vi "Mapping v10.6.1.vi"(5 "Simulate Spectra":bool, 7 "Simulate Drive":bool) -> ()   [LabVIEW 2010]
uses:
  TypeDefs/Mapping Spectra Params.ctl
  TypeDefs/Mapping Drive Params v10.6.0.ctl
  NPC3SG/TypeDefs/NPC3SG Set Positions.ctl
  NPC3SG/TypeDefs/NPC3SG Current Values.ctl
  iHR550/TypeDefs/iHR Current Values.ctl
  ITC503/TypeDefs/ITC503 Current Values.ctl
  TypeDefs/Mapping Input Parameters v10.6.0.ctl
  Symphony/TypeDefs/Symphony Area Format.ctl
  <vilib>/Utility/miscctls.llb/LVPointTypeDef.ctl
  Global Variables.vi
panel:
  in  "Input Parameters":T1={"Drive Connection Port"="", "ITC503 Current Values"={"ITC503 Heater"=0.0, "ITC503 Temperature"=0.0, "ITC503 P"=0.0, "ITC503 I"=0.0, "ITC503 D"=0.0, "ITC503 Setpoint"=0.0, "ITC503 Gradient"=0.0, "ITC503 Heater Auto"=FALSE, "ITC503 PID Auto"=FALSE}, "Wavelengths (nm)"=[], "Drive Current Values"={"Drive X Position"=0.0, "Drive Y Position"=0.0, "Drive Z Position"=0.0}, "iHR Current Values"={"iHR 550 Front Entrance"=0.0, "iHR550 Side Exit"=0.0, "iHR550 Wavelength"=897.9988, "iHR550 Exit Mirror"=2, "iHR550 Grating"="1", "Grating Index"=1}, "Spectra Settings"={"Integration Time"=1.0, "Repetitions"=1, "Mapping Spectra"=TRUE}, "CCD3500 Temperature"=0.0, "Simulate Drive"=FALSE, "Simulate Spectra"=FALSE, "JYCCDLib.IJYCCDReqd"=refnum, "CCD Area"={"XStart"=1, "YStart"=1, "XStop"=2048, "YStop"=512, "XBin"=1, "YBin"=1}, "CCD Gain"=1, "CCD ADC"=0} {"CCD ADC" items=["20 kHz       ", " 1 MHz       ", " 1 MHz Ultra ", "500 kHz Wrap"]; "CCD Gain" items=["High Light", "Best Dynamic Range", "High Sensitivity"]; "ITC503 Current Values"."ITC503 Gradient" format="%.2f"; "ITC503 Current Values"."ITC503 Setpoint" min=-273.0 max=300000.0 step=0.0001 format="%.1f"; "ITC503 Current Values"."ITC503 I" format="%_1f"; "ITC503 Current Values"."ITC503 P" format="%_1f"; "ITC503 Current Values"."ITC503 Temperature" min=0.0 max=1645.0 step=1e-05 format="%.2f"; "ITC503 Current Values"."ITC503 Heater" min=0.0 max=100.0 step=0.01 scale=0.0..100.0; "Drive Current Values"."Drive Z Position" min=-273.0 max=300000.0 step=0.0001 format="%.3f"; "Drive Current Values"."Drive Y Position" min=-273.0 max=300000.0 step=0.0001 format="%.3f"; "Drive Current Values"."Drive X Position" min=-273.0 max=300000.0 step=0.0001 format="%.3f"; "iHR Current Values"."iHR550 Exit Mirror" items=["EntranceMirror", "ExitMirror", "Front", "Side"]; "Spectra Settings"."Repetitions" min=1 max=100 step=1; "Spectra Settings"."Integration Time" min=0.5 max=6000.0 step=1.0 format="%.1f"}
  out "JYCCDLib.IJYCCDReqd":refnum<k7>
  out "AutoClose":bool
  out "ITC503 Temperature":dbl caption="Sample (K)" min=10.0 max=160.0 step=0.1 format="%.3f"
  out "CCD3500 Temperature":dbl caption="CCD (°C)" min=10.0 max=160.0 step=0.1 format="%.1f"
  in  "CCD Current Rep.":string="0/0"
  in  "Pause":bool
  out "Current Position":T3 {"Drive Z Position" min=-273.0 max=300000.0 step=0.0001 format="%.3f"; "Drive Y Position" min=-273.0 max=300000.0 step=0.0001 format="%.3f"; "Drive X Position" min=-273.0 max=300000.0 step=0.0001 format="%.3f"}
  out "Target Position":T7={"Drive X Set"=10.0, "Drive Y Set"=10.0, "Drive Z Set"=10.0} {"Drive X Set" min=10.0 max=160.0 step=0.1 format="%.3f"; "Drive Z Set" min=10.0 max=160.0 step=0.1 format="%.3f"; "Drive Y Set" min=10.0 max=160.0 step=0.1 format="%.3f"}
  out "Progress":u8(slide) max=10 scale=0.0..100.0
  out "Objective Running":bool caption="Obj."
  out "CCD Running":bool caption="CCD"
  in  "Save Map":bool
  in  "Spectra Params":T5={"Integration Time"=10.0, "Repetitions"=10, "Mapping Spectra"=TRUE} {"Repetitions" min=1 max=100 step=1; "Integration Time" min=0.5 max=6000.0 step=1.0 format="%.1f"}
  in  "Drive Settings":refnum<visa-resource-name>
  in  "Z Position":dbl caption="Z (µm)" min=0.0 max=100.0 step=0.1 format="%.1f"
  in  "Mapping Params":T8={"X Start Position"=0.0, "X Stop Position"=10.0, "Y Start Position"=0.0, "Y Stop Position"=10.0, "Step Size"=1.0} {"Step Size" min=0.005 max=20.0 step=0.005 format="%.3f"; "Y Stop Position" min=0.0 max=140.0 step=0.005 format="%.3f"; "Y Start Position" min=0.0 max=140.0 step=0.005 format="%.3f"; "X Stop Position" min=0.0 max=140.0 step=0.005 format="%.3f"; "X Start Position" min=0.0 max=140.0 step=0.005 format="%.3f"}
  in  "Exit":bool
  out "Measuring":bool
  in  "Start":bool
  out "Filename":string
  out "Full Data":dbl[][](array[numeric])
  out "Live Data":dbl[][](array[numeric])
  in  "ITC503 Current Values":T2 {"ITC503 Gradient" format="%.2f"; "ITC503 Setpoint" min=-273.0 max=300000.0 step=0.0001 format="%.1f"; "ITC503 I" format="%_1f"; "ITC503 P" format="%_1f"; "ITC503 Temperature" min=0.0 max=1645.0 step=1e-05 format="%.2f"; "ITC503 Heater" min=0.0 max=100.0 step=0.01 scale=0.0..100.0}
  in  "iHR Current Values":T4={"iHR 550 Front Entrance"=0.0, "iHR550 Side Exit"=0.0, "iHR550 Wavelength"=897.9988, "iHR550 Exit Mirror"=2, "iHR550 Grating"="1", "Grating Index"=1} {"iHR550 Exit Mirror" items=["EntranceMirror", "ExitMirror", "Front", "Side"]}
  in  "Wavelengths (nm)":dbl[](array[numeric])
  # "Status"
  # "Active"
  # "Target"
  # "Current"
  # "Parameters"
  # "Spectral"
  # "Spectral / Video Mapping"
  # "Mapping"
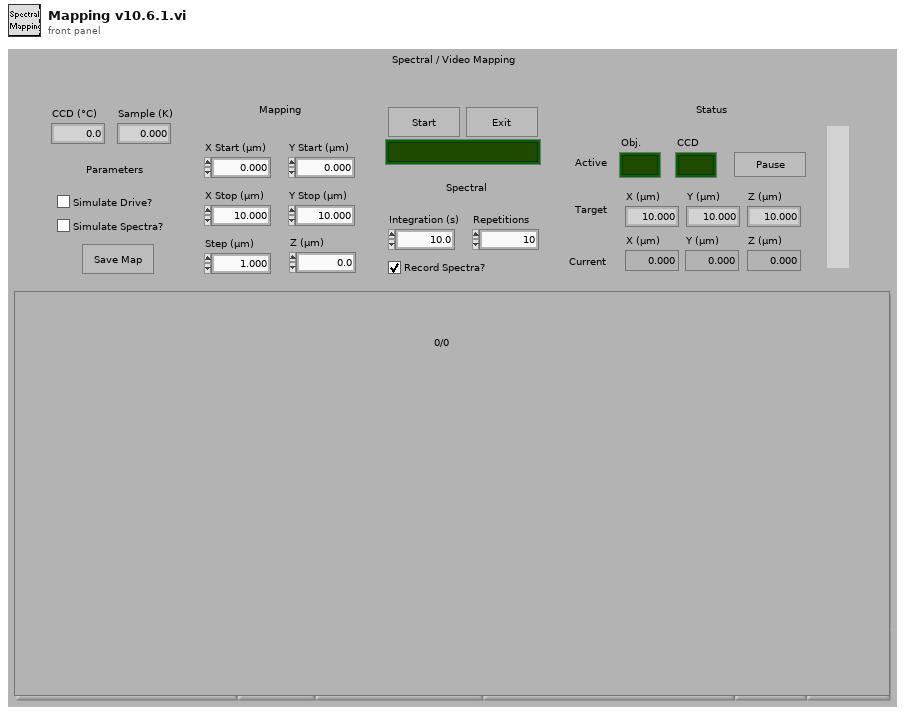
[diagram p1: front panel]
types:
  T1 = typedef "Mapping Input Parameters v10.6.0.ctl" = cluster{"Drive Connection Port":refnum<visa-resource-name>, "ITC503 Current Values":T2, "Wavelengths (nm)":dbl[], "Drive Current Values":T3, "iHR Current Values":T4, "Spectra Settings":T5, "CCD3500 Temperature":dbl, "Simulate Drive":bool, "Simulate Spectra":bool, "JYCCDLib.IJYCCDReqd":refnum<k7>, "CCD Area":T6, "CCD Gain":u16, "CCD ADC":u16}
  T2 = typedef "ITC503 Current Values.ctl" = cluster{"ITC503 Heater":dbl, "ITC503 Temperature":dbl, "ITC503 P":dbl, "ITC503 I":dbl, "ITC503 D":dbl, "ITC503 Setpoint":dbl, "ITC503 Gradient":dbl, "ITC503 Heater Auto":bool, "ITC503 PID Auto":bool}
  T3 = typedef "NPC3SG Current Values.ctl" = cluster{"Drive X Position":dbl, "Drive Y Position":dbl, "Drive Z Position":dbl}
  T4 = typedef "iHR Current Values.ctl" = cluster{"iHR 550 Front Entrance":dbl, "iHR550 Side Exit":dbl, "iHR550 Wavelength":dbl, "iHR550 Exit Mirror":i32, "iHR550 Grating":string, "Grating Index":i32}
  T5 = typedef "Mapping Spectra Params.ctl" = cluster{"Integration Time":dbl, "Repetitions":u16, "Mapping Spectra":bool}
  T6 = typedef "Symphony Area Format.ctl" = cluster{"XStart":i32, "YStart":i32, "XStop":i32, "YStop":i32, "XBin":i32, "YBin":i32}
  T7 = typedef "NPC3SG Set Positions.ctl" = cluster{"Drive X Set":dbl, "Drive Y Set":dbl, "Drive Z Set":dbl}
  T8 = typedef "Mapping Drive Params v10.6.0.ctl" = cluster{"X Start Position":dbl, "X Stop Position":dbl, "Y Start Position":dbl, "Y Stop Position":dbl, "Step Size":dbl}
  T9 = typedef "LVPointTypeDef.ctl" = cluster{"Horizontal":i16, "Vertical":i16}
  T10 = cluster{"Intensities":dbl[], "Wavelengths":dbl[]}[]
  T11 = cluster{"Intensities":dbl[], "Wavelengths":dbl[]}
  T12 = enum32{"invalid app kind", "Development System", "Run Time System", "Student Edition", "Embedded LabVIEW", "Evaluation", "Custom"}
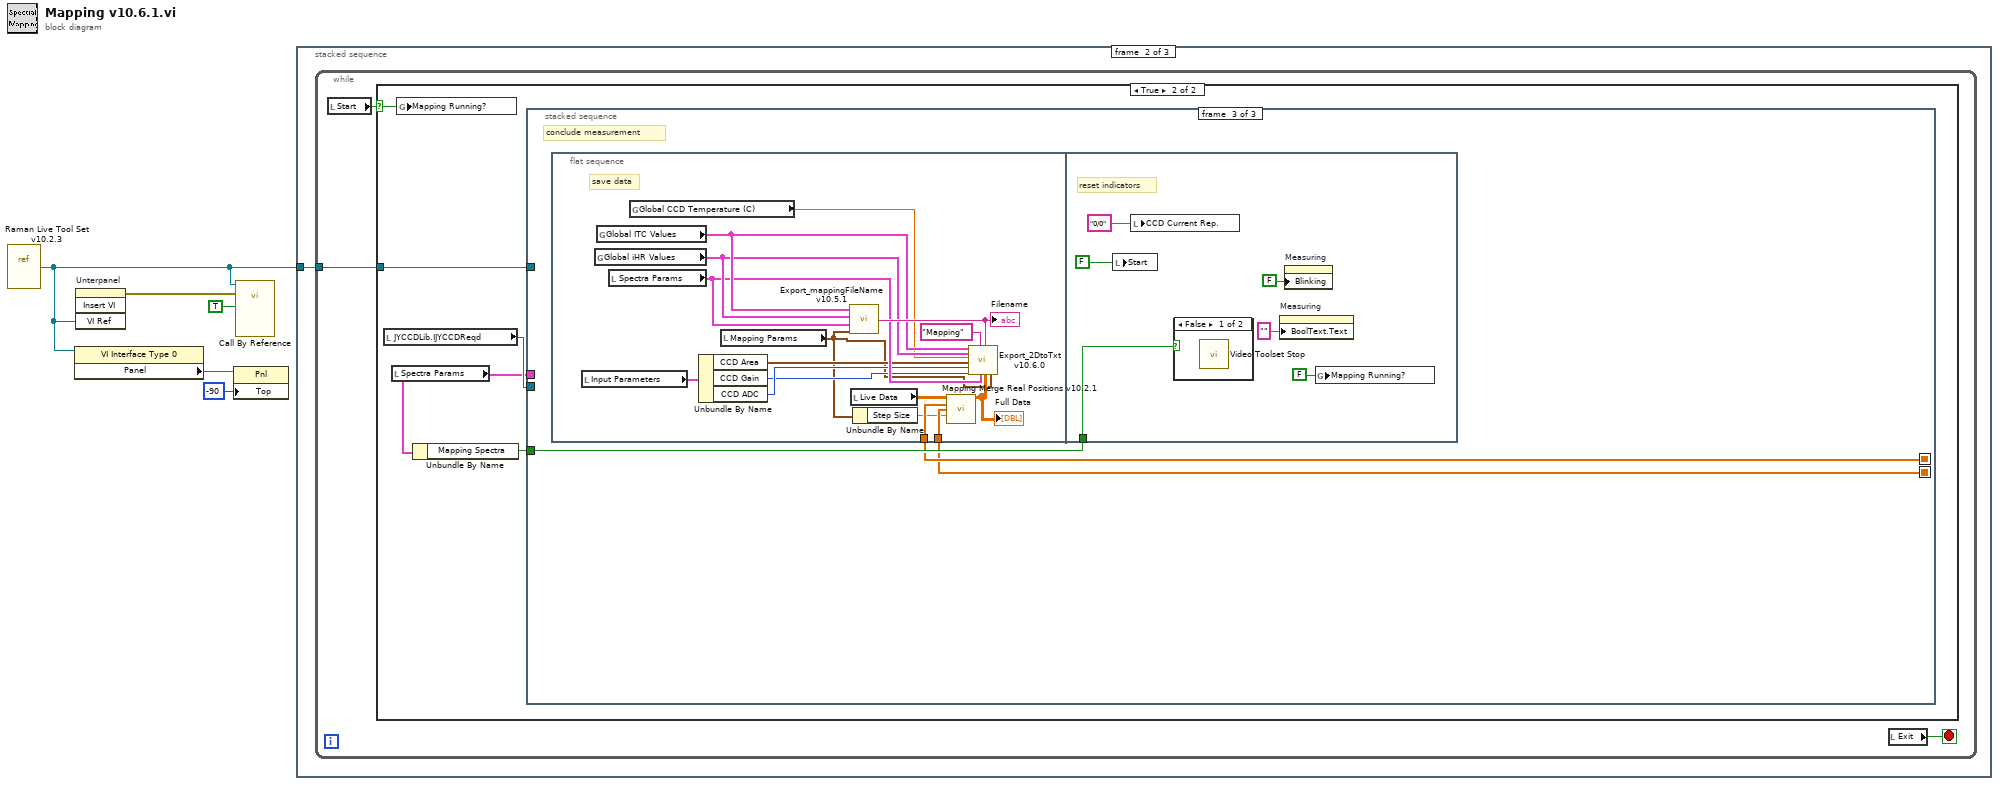
[diagram p0: block diagram]
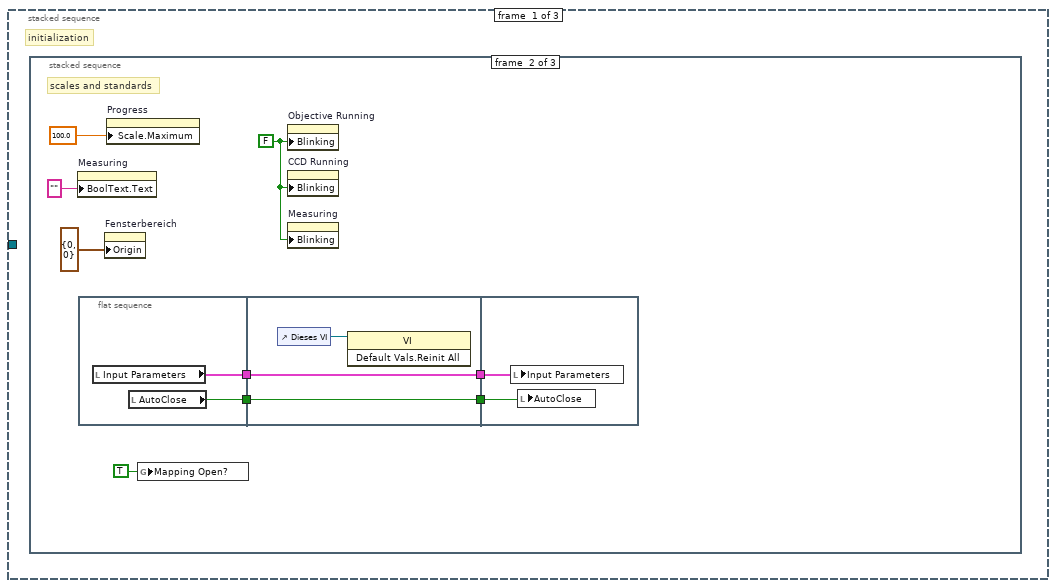
[diagram p2: hidden frame]
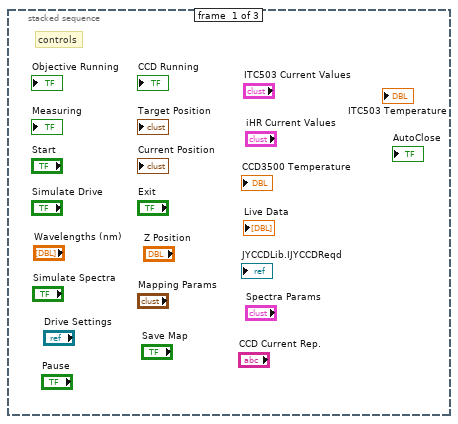
[diagram p3: hidden frame]
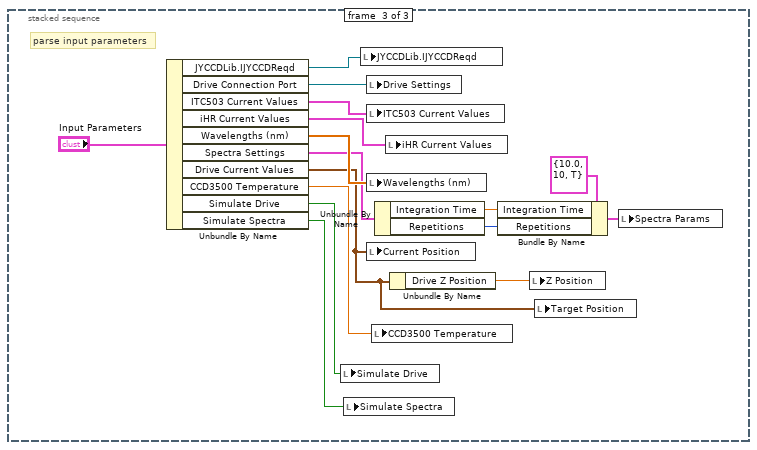
[diagram p4: hidden frame]
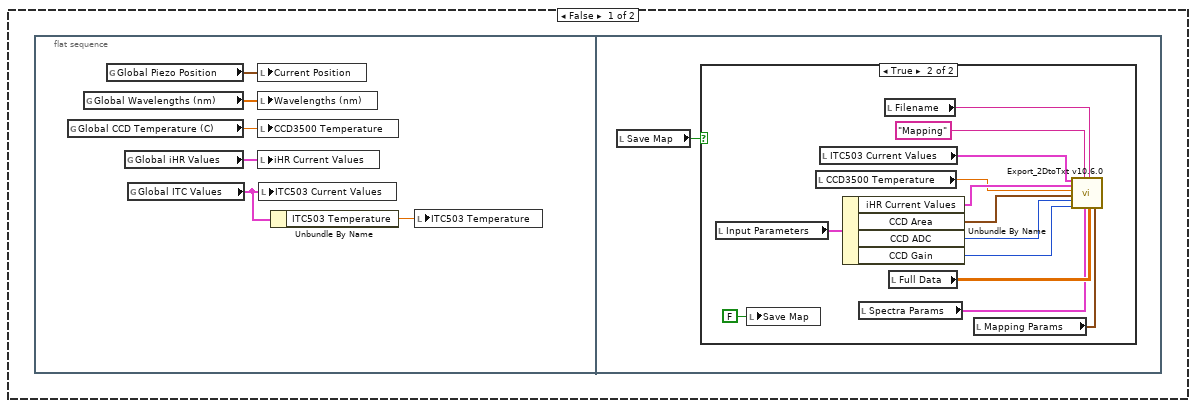
[diagram p5: hidden frame]
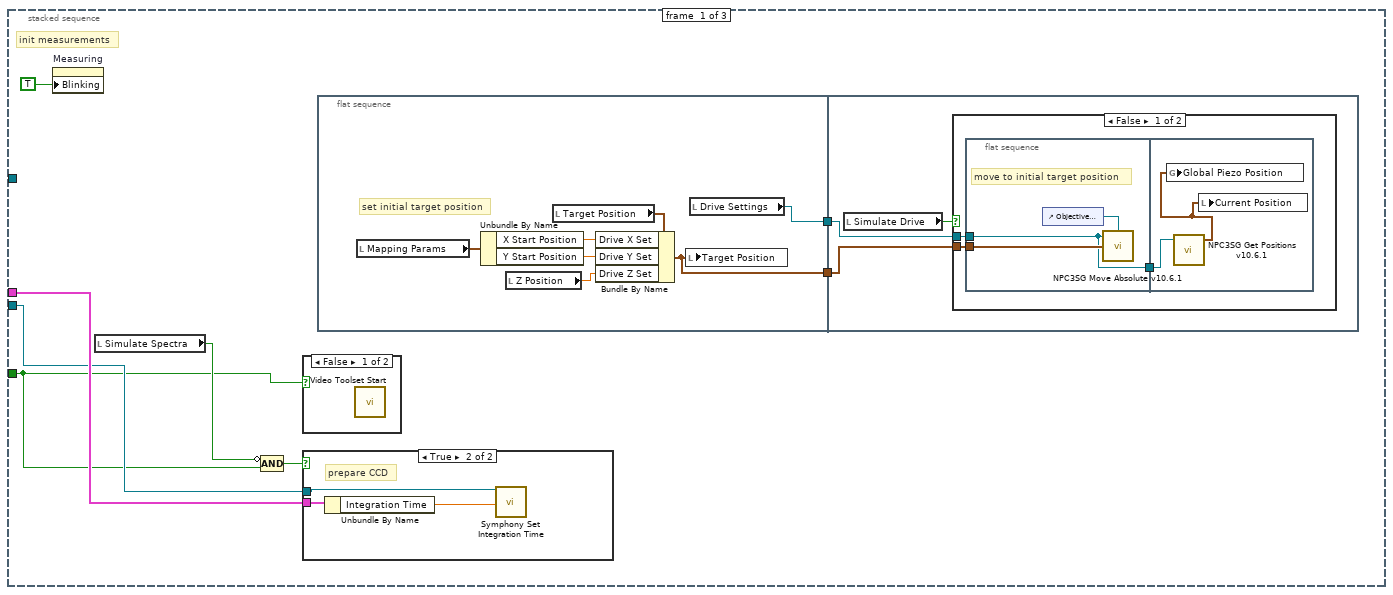
[diagram p7: hidden frame]
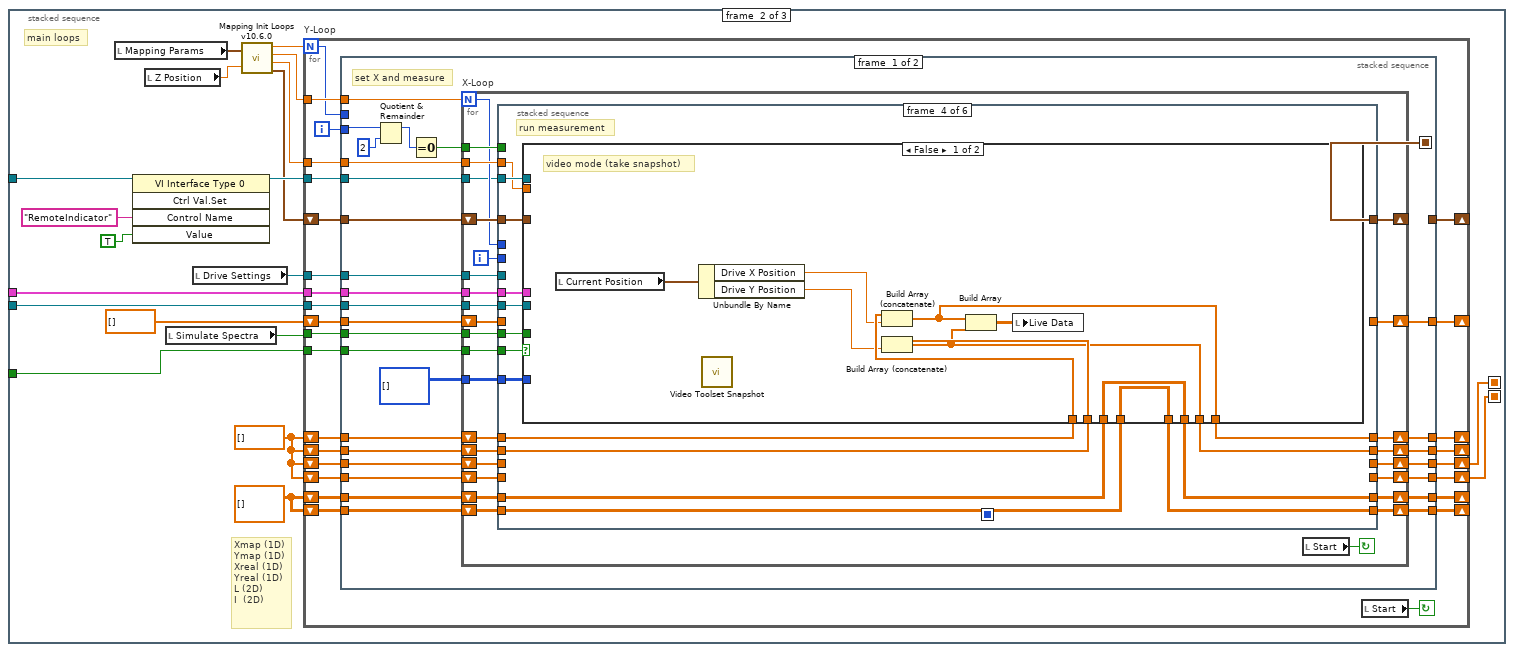
[diagram p11: hidden frame]
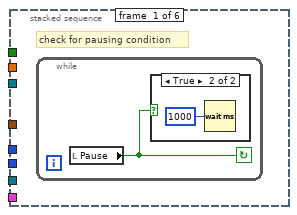
[diagram p12: hidden frame]
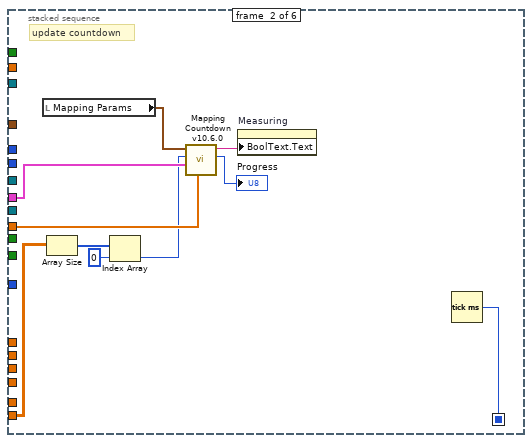
[diagram p14: hidden frame]
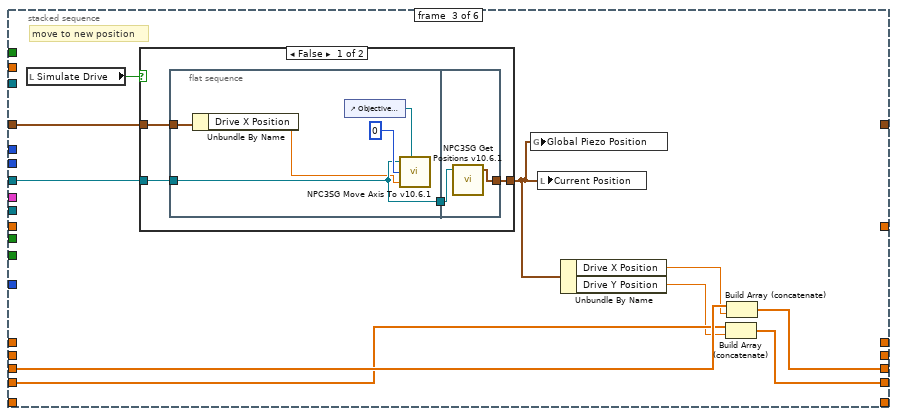
[diagram p15: hidden frame]
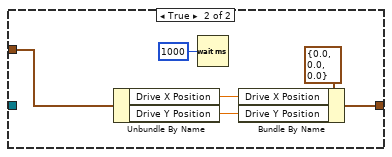
[diagram p16: hidden frame]
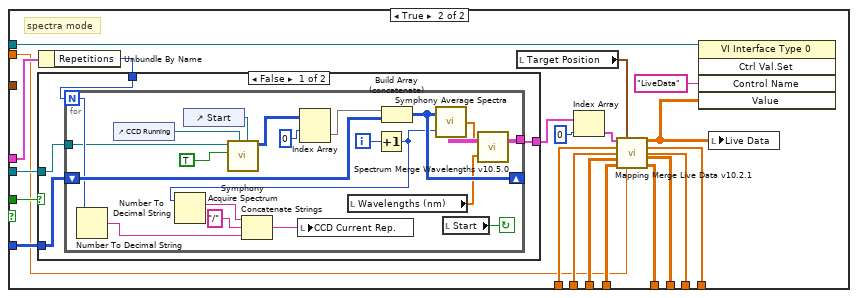
[diagram p17: hidden frame]
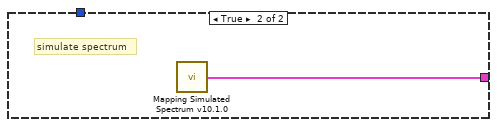
[diagram p18: hidden frame]
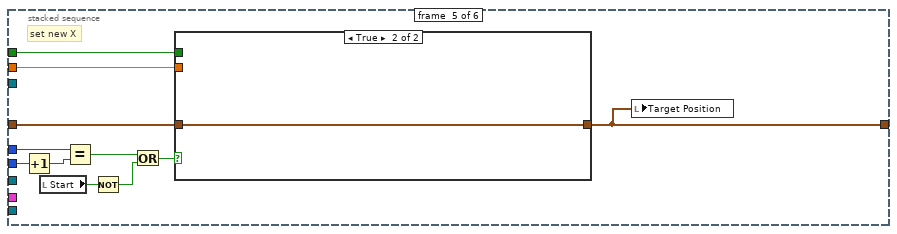
[diagram p19: hidden frame]
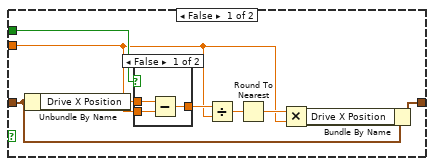
[diagram p20: hidden frame]
diagram:
  n1 = vi-ref "Raman Live Tool Set v10.2.3.vi"() -> (w3:refnum<vi>)
  n2 = property class="VI Interface Type 0"(reference=w3) -> ("Panel"=w2:refnum<vi>)  [unwired: 1 in, 2 out]
  n3 = invoke on="Unterpanel" class="Unterpanel" method="Insert VI"("VI Ref"=w3) -> (error out=w5:errorcluster)  [unwired: 3 in, 3 out]
  n4 = property class="Pnl"(reference=w2, "Top"=-90 ("Position:Oben")) -> ()  [unwired: 1 in, 2 out]
  n5 = call-by-ref "?"(reference=w3, error in=w5, "RemoteIndicator"=TRUE) -> ()  [unwired: 3 in, 2 out]
  n6 = stacked-sequence {
    tunnel: w3 -> [_ w38 w403]
    frame #0 {
      # "initialization"
      n7 = stacked-sequence {
        frame #0 {
          # "controls"
        }
        frame #1 {
          w12 = FALSE ("Blinkend")
          # "scales and standards"
          n8 = property on="Measuring" class="Bool (strict)"("BoolText.Text"="" ("Boolescher Text.Text")) -> ()  [unwired: 2 in, 2 out]
          n9 = flat-sequence {
            tunnel: [w16] -> w9
            tunnel: [w15] -> w6
            tunnel: [w18] -> w10
            tunnel: w9 -> [w18]
            tunnel: [w17] -> w7
            tunnel: w6 -> [w17]
            tunnel: w10 -> [w21]
            tunnel: w7 -> [w20]
            frame #0 {
              n10 = local read "Input Parameters"() -> (w16:T1)
              n11 = local read "AutoClose"() -> (w15:bool)
            }
            frame #1 {
              n12 = control-ref of="Dieses VI"() -> (w19:refnum<vi>)
              n13 = invoke class="VI" method="Default Vals.Reinit All"(reference=w19) -> ()  [unwired: 2 in, 3 out]
            }
            frame #2 {
              n14 = local write "Input Parameters"(w21) -> ()
              n15 = local write "AutoClose"(w20) -> ()
            }
          }
          n16 = property on="Fensterbereich" class="Pane"("Origin"=T9 {"Horizontal"=0, "Vertical"=0}) -> ()  [unwired: 2 in, 2 out]
          n17 = property on="Progress" class="Slide (strict)"("Scale.Maximum"=100.0 ("Skalierung.Bereich:Maximum")) -> ()  [unwired: 2 in, 2 out]
          n18 = global write "Global Variables.vi" "Mapping Open?"(TRUE ("Mapping Open?")) -> ()
          n19 = property on="Objective Running" class="Bool (strict)"("Blinking"=w12) -> ()  [unwired: 2 in, 2 out]
          n20 = property on="CCD Running" class="Bool (strict)"("Blinking"=w12) -> ()  [unwired: 2 in, 2 out]
          n21 = property on="Measuring" class="Bool (strict)"("Blinking"=w12) -> ()  [unwired: 2 in, 2 out]
        }
        frame #2 {
          # "parse input parameters"
          n22 = Unbundle By Name("Input Parameters") -> ("JYCCDLib.IJYCCDReqd"=w24:refnum<k7>, "Drive Connection Port"=w36:refnum<visa-resource-name>, "ITC503 Current Values"=w37:T2, "iHR Current Values"=w27:T4, "Wavelengths (nm)"=w35:dbl[], "Spectra Settings"=w33:T5, "Drive Current Values"=w22:T3, "CCD3500 Temperature"=w28:dbl, "Simulate Drive"=w26:bool, "Simulate Spectra"=w25:bool)
          n23 = local write "Simulate Drive"(w26) -> ()
          n24 = local write "Simulate Spectra"(w25) -> ()
          n25 = local write "JYCCDLib.IJYCCDReqd"(w24) -> ()
          n26 = local write "Drive Settings"(w36) -> ()
          n27 = local write "ITC503 Current Values"(w37) -> ()
          n28 = local write "Wavelengths (nm)"(w35) -> ()
          n29 = local write "Current Position"(w22) -> ()
          n30 = local write "CCD3500 Temperature"(w28) -> ()
          n31 = Unbundle By Name(w33) -> ("Integration Time"=w31:dbl, "Repetitions"=w30:u16)
          n32 = local write "iHR Current Values"(w27) -> ()
          n33 = Unbundle By Name(w22) -> ("Drive Z Position"=w34:dbl)
          n34 = Bundle By Name(cluster=T5 {"Integration Time"=10.0, "Repetitions"=10, "Mapping Spectra"=TRUE} ("Mapping Spectra Settings"), "Integration Time"=w31, "Repetitions"=w30) -> (w29:T5)
          n35 = local write "Z Position"(w34) -> ()
          n36 = local write "Target Position"(w22) -> ()
          n37 = local write "Spectra Params"(w29) -> ()
        }
      }
    }
    frame #1 {
      n38 = while {
        tunnel: w38 -> [w41]
        stop <- w40 stop-if-true
        n39 = local read "Start"() -> (w39:bool)
        n40 = case shown="True" w39 {
          selector: w39 -> [_ w63]
          tunnel: w41 -> [_ w66]
          frame False {
            n41 = flat-sequence {
              frame #0 {
                n42 = global read "Global Variables.vi" "Global CCD Temperature (C)"() -> (w47:dbl)
                n43 = global read "Global Variables.vi" "Global Wavelengths (nm)"() -> (w45:dbl[])
                n44 = global read "Global Variables.vi" "Global Piezo Position"() -> (w46:T3)
                n45 = global read "Global Variables.vi" "Global iHR Values"() -> (w44:T4)
                n46 = global read "Global Variables.vi" "Global ITC Values"() -> (w43:T2)
                n47 = local write "Current Position"(w46) -> ()
                n48 = local write "Wavelengths (nm)"(w45) -> ()
                n49 = local write "CCD3500 Temperature"(w47) -> ()
                n50 = local write "iHR Current Values"(w44) -> ()
                n51 = local write "ITC503 Current Values"(w43) -> ()
                n52 = Unbundle By Name(w43) -> ("ITC503 Temperature"=w42:dbl)
                n53 = local write "ITC503 Temperature"(w42) -> ()
              }
              frame #1 {
                n54 = local read "Save Map"() -> (w48:bool)
                n55 = case shown="True" w48 {
                  frame False {
                  }
                  frame True {
                    n56 = local read "Input Parameters"() -> (w57:T1)
                    n57 = local write "Save Map"(FALSE ("Save Map")) -> ()
                    n58 = local read "CCD3500 Temperature"() -> (w51:dbl)
                    n59 = local read "ITC503 Current Values"() -> (w54:T2)
                    n60 = Unbundle By Name(w57) -> ("iHR Current Values"=w52:T4, "CCD Area"=w53:T6, "CCD ADC"=w56:u16, "CCD Gain"=w55:u16)
                    n61 = local read "Spectra Params"() -> (w50:T5)
                    n62 = local read "Filename"() -> (w60:string)
                    n63 = local read "Full Data"() -> (w58:dbl[][])
                    n64 = local read "Mapping Params"() -> (w49:T8)
                    n65 = call "Export_2DtoTxt v10.6.0.vi"("ITC503 Current Values"=w54, "iHR Current Values"=w52, "CCD Temperature"=w51, "CCD Area"=w53, "CCD ADC"=w56, "CCD Gain"=w55, "Export Type"="Mapping", "Spectra Settings"=w50, "Filename"=w60, "Data (2D)"=w58, "Mapping Parameters"=w49) -> ()  [unwired: 8 in, 1 out]
                  }
                }
              }
            }
          }
          frame True {
            n66 = local read "JYCCDLib.IJYCCDReqd"() -> (w65:refnum<k7>)
            n67 = local read "Spectra Params"() -> (w64:T5)
            n68 = global write "Global Variables.vi" "Mapping Running?"(w63) -> ()
            n69 = Unbundle By Name(w64) -> ("Mapping Spectra"=w62:bool)
            n70 = stacked-sequence {
              seq-local: [_ w96 _] -> [_ _ w378]
              seq-local: [_ w97 _] -> [_ _ w377]
              tunnel: w66 -> [_ w107 _]
              tunnel: w62 -> [w67 w106 w379]
              tunnel: w64 -> [w69 w104 _]
              tunnel: w65 -> [w68 w103 _]
              frame #0 {
                # "init measurements"
                n71 = property on="Measuring" class="Bool (strict)"("Blinking"=TRUE ("Blinkend")) -> ()  [unwired: 2 in, 2 out]
                n72 = local read "Simulate Spectra"() -> (w71:bool)
                n73 = Compound Arithmetic op=AND(invert w71, w67) -> (w70:bool)
                n74 = case shown="False" w67 {
                  frame False {
                    n75 = call "Video Toolset Start.vi"() -> ()  [unwired: 3 in]
                  }
                  frame True {
                  }
                }
                n76 = case shown="True" w70 {
                  tunnel: w68 -> [_ w77]
                  tunnel: w69 -> [_ w76]
                  frame False {
                  }
                  frame True {
                    # "prepare CCD"
                    n77 = Unbundle By Name(w76) -> ("Integration Time"=w75:dbl)
                    n78 = call "Symphony Set Integration Time.vi"("JYCCDLib.IJYCCDReqd"=w77, "Integration (s)"=w75) -> ()  [unwired: 13 in, 1 out]
                  }
                }
                n79 = flat-sequence {
                  tunnel: [w79] -> w73
                  tunnel: [w78] -> w72
                  tunnel: w73 -> [w85]
                  tunnel: w72 -> [w86]
                  frame #0 {
                    # "set initial target position"
                    n80 = local read "Mapping Params"() -> (w84:T8)
                    n81 = Unbundle By Name(w84) -> ("X Start Position"=w82:dbl, "Y Start Position"=w81:dbl)
                    n82 = local read "Z Position"() -> (w80:dbl)
                    n83 = local read "Target Position"() -> (w83:T7)
                    n84 = Bundle By Name(cluster=w83, "Drive X Set"=w82, "Drive Y Set"=w81, "Drive Z Set"=w80) -> (w79:T7)
                    n85 = local write "Target Position"(w79) -> ()
                    n86 = local read "Drive Settings"() -> (w78:refnum<visa-resource-name>)
                  }
                  frame #1 {
                    n87 = local read "Simulate Drive"() -> (w87:bool)
                    n88 = case shown="False" w87 {
                      tunnel: w86 -> [w90 _]
                      tunnel: w85 -> [w88 _]
                      frame False {
                        n89 = flat-sequence {
                          tunnel: w90 -> [w91]
                          tunnel: [w91] -> w89
                          tunnel: w88 -> [w92]
                          tunnel: w89 -> [w94]
                          frame #0 {
                            # "move to initial target position"
                            n90 = control-ref of="Objective Running"() -> (w93:refnum<vi>)
                            n91 = call "NPC3SG Move Absolute v10.6.1.vi"("Running"=w93, "Drive New Abs. Positions"=w92, "Drive Visa Name"=w91) -> ()  [unwired: 2 in]
                          }
                          frame #1 {
                            n92 = call "NPC3SG Get Positions v10.6.1.vi"("Drive Visa Name"=w94) -> ("Drive Current Values"=w95:T3)  [unwired: 6 in]
                            n93 = global write "Global Variables.vi" "Global Piezo Position"(w95) -> ()
                            n94 = local write "Current Position"(w95) -> ()
                          }
                        }
                      }
                      frame True {
                      }
                    }
                  }
                }
              }
              frame #1 {
                w115 = dbl[][] []
                w98 = dbl[] []
                # "main loops"
                # "Xmap (1D)\nYmap (1D)\nXreal (1D)\nYreal (1D)\nL (2D)\nI  (2D)"
                n95 = local read "Mapping Params"() -> (w101:T8)
                n96 = invoke class="VI Interface Type 0" method="Ctrl Val.Set"(reference=w107, "Control Name"="RemoteIndicator" ("Elementname"), "Value"=TRUE) -> (reference out=w109:refnum<vi>)  [unwired: 2 in, 4 out]
                n97 = local read "Z Position"() -> (w100:dbl)
                n98 = local read "Simulate Spectra"() -> (w99:bool)
                n99 = local read "Drive Settings"() -> (w102:refnum<visa-resource-name>)
                n100 = call "Mapping Init Loops v10.6.0.vi"("Z Position"=w100, "Mapping Params"=w101) -> ("Start Positions"=w108:T3, "Step Size"=w110:dbl, "X Steps"=w111:dbl, "Y Steps"=w112:dbl)
                n101 = for "Y-Loop" {
                  N: w112 -> [w128]
                  tunnel: w111 -> [w141]
                  tunnel: w110 -> [w140]
                  shift-right: [w126] -> _
                  shift-left: w108 -> [w127]
                  shift-right: [w132] -> _
                  shift-left: w115 -> [w136]
                  shift-right: [w133] -> _
                  shift-left: w115 -> [w137]
                  shift-right: [w135] -> _
                  shift-left: w98 -> [w139]
                  shift-right: [w134] -> _
                  shift-left: w98 -> [w138]
                  tunnel: w109 -> [w130]
                  tunnel: w99 -> [w129]
                  tunnel: w102 -> [w125]
                  tunnel: w106 -> [w124]
                  tunnel: w104 -> [w123]
                  shift-right: [w121] -> _
                  shift-left: dbl[] [] -> [w122]
                  tunnel: w103 -> [w120]
                  shift-right: [w117] -> w97
                  shift-left: w98 -> [w118]
                  shift-right: [w116] -> w96
                  shift-left: w98 -> [w119]
                  i -> [w131]
                  stop <- w142 continue-if-true
                  n102 = stacked-sequence {
                    seq-local: [w156 _] -> [_ w352]
                    tunnel: w141 -> [w171 _]
                    tunnel: w140 -> [w170 w353]
                    tunnel: w139 -> [w169 _]
                    tunnel: w138 -> [w168 _]
                    tunnel: w137 -> [w167 _]
                    tunnel: w136 -> [w143 _]
                    tunnel: [w166 _] -> w135
                    tunnel: [w165 _] -> w134
                    tunnel: [w164 _] -> w133
                    tunnel: [w163 _] -> w132
                    tunnel: w131 -> [w160 w356]
                    tunnel: w130 -> [w158 _]
                    tunnel: w129 -> [w157 _]
                    tunnel: w128 -> [_ w354]
                    tunnel: w127 -> [w155 _]
                    tunnel: [_ w350] -> w126
                    tunnel: w125 -> [w154 w351]
                    tunnel: w124 -> [w153 _]
                    tunnel: w123 -> [w152 _]
                    tunnel: w122 -> [w151 _]
                    tunnel: [w150 _] -> w121
                    tunnel: w120 -> [w149 _]
                    tunnel: w119 -> [w147 _]
                    tunnel: w118 -> [w146 _]
                    tunnel: [w145 _] -> w117
                    tunnel: [w144 _] -> w116
                    frame #0 {
                      # "set X and measure"
                      n103 = Quotient & Remainder(x=w160, y=2) -> (x-y*floor(x/y)=w161:i32)  [unwired: 1 out]
                      n104 = Equal To 0?(x=w161) -> (x = 0?=w159:bool)
                      n105 = for "X-Loop" {
                        N: w171 -> [w185]
                        tunnel: w170 -> [w197]
                        shift-right: [w196] -> w156
                        shift-left: w155 -> [w198]
                        shift-right: [w191] -> w166
                        shift-left: w169 -> [w195]
                        shift-right: [w190] -> w165
                        shift-left: w168 -> [w194]
                        shift-right: [w188] -> w164
                        shift-left: w167 -> [w193]
                        shift-right: [w189] -> w163
                        shift-left: w143 -> [w192]
                        tunnel: w159 -> [w187]
                        tunnel: w158 -> [w184]
                        tunnel: w157 -> [w183]
                        tunnel: w154 -> [w182]
                        tunnel: w153 -> [w181]
                        tunnel: w152 -> [w180]
                        shift-right: [w179] -> w150
                        shift-left: w151 -> [w178]
                        tunnel: w149 -> [w177]
                        tunnel: u16[][] [] -> [w176]
                        shift-right: [w172] -> w144
                        shift-left: w147 -> [w175]
                        shift-right: [w173] -> w145
                        shift-left: w146 -> [w174]
                        i -> [w186]
                        stop <- w199 continue-if-true
                        n106 = stacked-sequence {
                          seq-local: [_ w206 _ _ _ _] -> [_ _ _ _ _ w341]
                          tunnel: w198 -> [_ _ w221 w254 w318 _]
                          tunnel: w197 -> [_ _ _ w239 w316 _]
                          tunnel: [_ _ _ _ w315 _] -> w196
                          tunnel: w195 -> [_ _ _ w253 _ _]
                          tunnel: w194 -> [_ _ _ w252 _ _]
                          tunnel: w193 -> [_ _ _ w250 _ _]
                          tunnel: w192 -> [_ w205 _ w251 _ _]
                          tunnel: [_ _ _ w249 _ _] -> w191
                          tunnel: [_ _ _ w248 _ _] -> w190
                          tunnel: [_ _ _ w247 _ _] -> w189
                          tunnel: [_ _ _ w246 _ _] -> w188
                          tunnel: w187 -> [_ _ _ _ w317 _]
                          tunnel: w186 -> [_ _ _ _ w321 _]
                          tunnel: w185 -> [_ _ _ _ w319 _]
                          tunnel: w184 -> [_ _ _ w245 _ _]
                          tunnel: w183 -> [_ _ _ w244 _ _]
                          tunnel: w182 -> [_ _ w219 _ _ _]
                          tunnel: w181 -> [_ _ _ w243 _ _]
                          tunnel: w180 -> [_ w208 _ w241 _ _]
                          tunnel: [_ _ _ _ _ w338] -> w179
                          tunnel: w178 -> [_ w207 _ _ _ w340]
                          tunnel: w177 -> [_ _ _ w242 _ _]
                          tunnel: w176 -> [_ _ _ w240 _ _]
                          tunnel: w175 -> [_ _ w218 _ _ _]
                          tunnel: w174 -> [_ _ w217 _ _ _]
                          tunnel: [_ _ w214 _ _ _] -> w173
                          tunnel: [_ _ w213 _ _ _] -> w172
                          frame #0 {
                            # "check for pausing condition"
                            n107 = while {
                              stop <- w200 continue-if-true
                              n108 = local read "Pause"() -> (w200:bool)
                              n109 = case shown="True" w200 {
                                frame False {
                                }
                                frame True {
                                n110 = Wait (ms)(milliseconds to wait=u32 1000) -> ()  [unwired: 1 out]
                                }
                              }
                            }
                          }
                          frame #1 {
                            # "update countdown"
                            n111 = local read "Mapping Params"() -> (w211:T8)
                            n112 = Array Size(array=w205) -> (size(s)=w204:i32[])
                            n113 = Index Array(array=w204, index=0) -> (element=w202:i32)
                            n114 = call "Mapping Countdown v10.6.0.vi"("Execution Times (s)"=w207, "Mapping Spectra Settings"=w208, "Ready Steps"=w202, "Mapping Drive Parameters"=w211) -> ("Progress"=→"Progress":i16, "Time String"=w209:string)  [unwired: 6 in]
                            n115 = property on="Measuring" class="Bool (strict)"("BoolText.Text"=w209) -> ()  [unwired: 2 in, 2 out]
                            n116 = Tick Count (ms)() -> (millisecond timer value=w206:u32)
                          }
                          frame #2 {
                            # "move to new position"
                            n117 = local read "Simulate Drive"() -> (w220:bool)
                            n118 = case shown="False" w220 {
                              tunnel: w221 -> [w225 w237]
                              tunnel: w219 -> [w224 _]
                              tunnel: [w222 w233] -> w212
                              frame False {
                                n119 = flat-sequence {
                                tunnel: w225 -> [w227]
                                tunnel: w224 -> [w228]
                                tunnel: [w228] -> w223
                                tunnel: w223 -> [w232]
                                tunnel: [w231] -> w222
                                frame #0 {
                                n120 = Unbundle By Name(w227) -> ("Drive X Position"=w226:dbl)
                                n121 = control-ref of="Objective Running"() -> (w229:refnum<vi>)
                                n122 = call "NPC3SG Move Axis To v10.6.1.vi"("Drive Visa Name"=w228, "Running"=w229, "Axis"=0, "Drive Set"=w226) -> ()  [unwired: 3 in, 1 out]
                                }
                                frame #1 {
                                n123 = call "NPC3SG Get Positions v10.6.1.vi"("Drive Visa Name"=w232) -> ("Drive Current Values"=w231:T3)  [unwired: 6 in]
                                }
                                }
                              }
                              frame True {
                                n124 = Unbundle By Name(w237) -> ("Drive X Position"=w238:dbl, "Drive Y Position"=w235:dbl)
                                n125 = Wait (ms)(milliseconds to wait=u32 1000 ("Zu wartende ms")) -> ()  [unwired: 1 out]
                                n126 = Bundle By Name(cluster=T3 {"Drive X Position"=0.0, "Drive Y Position"=0.0, "Drive Z Position"=0.0} ("Drive Current Values"), "Drive X Position"=w238, "Drive Y Position"=w235) -> (w233:T3)
                              }
                            }
                            n127 = global write "Global Variables.vi" "Global Piezo Position"(w212) -> ()
                            n128 = local write "Current Position"(w212) -> ()
                            n129 = Unbundle By Name(w212) -> ("Drive X Position"=w216:dbl, "Drive Y Position"=w215:dbl)
                            n130 = Build Array (concatenate)(w217, w215) -> (w214:dbl[])
                            n131 = Build Array (concatenate)(w218, w216) -> (w213:dbl[])
                          }
                          frame #3 {
                            # "run measurement"
                            n132 = case shown="False" w243 {
                              tunnel: w254 -> [_ _]
                              tunnel: w253 -> [w261 w282]
                              tunnel: w252 -> [w260 w281]
                              tunnel: w251 -> [w263 w279]
                              tunnel: w250 -> [w264 w280]
                              tunnel: [w258 w276] -> w249
                              tunnel: [w259 w275] -> w248
                              tunnel: [w263 w278] -> w247
                              tunnel: [w264 w277] -> w246
                              tunnel: w245 -> [_ w284]
                              tunnel: w244 -> [_ w283]
                              tunnel: w242 -> [_ w272]
                              tunnel: w241 -> [_ w271]
                              tunnel: w240 -> [_ w269]
                              tunnel: w239 -> [_ w265]
                              frame False {
                                # "video mode (take snapshot)"
                                n133 = local read "Current Position"() -> (w262:T3)
                                n134 = Unbundle By Name(w262) -> ("Drive X Position"=w257:dbl, "Drive Y Position"=w256:dbl)
                                n135 = call "Video Toolset Snapshot.vi"() -> ()  [unwired: 12 in]
                                n136 = Build Array (concatenate)(w261, w257) -> (w258:dbl[])
                                n137 = Build Array (concatenate)(w260, w256) -> (w259:dbl[])
                                n138 = Build Array(w258, w259) -> (w255:dbl[][])
                                n139 = local write "Live Data"(w255) -> ()
                              }
                              frame True {
                                # "spectra mode"
                                n140 = Unbundle By Name(w271) -> ("Repetitions"=w270:u16)
                                n141 = case shown="False" w283 {
                                tunnel: [w288 w310] -> w268
                                tunnel: w272 -> [w289 _]
                                tunnel: w270 -> [w287 _]
                                tunnel: w269 -> [w286 _]
                                frame False {
                                n142 = for {
                                N: w287 -> [w296]
                                shift-right: [w307] -> _
                                shift-left: w286 -> [w308]
                                tunnel: [w305] -> w288
                                tunnel: w289 -> [w294]
                                i -> [w309]
                                stop <- w303 continue-if-true
                                n143 = Number To Decimal String(number=w296) -> (decimal integer string=w299:string)  [unwired: 1 in]
                                n144 = control-ref of="CCD Running"() -> (w302:refnum<vi>)
                                n145 = control-ref of="Start"() -> (w301:refnum<vi>)
                                n146 = call "Symphony Acquire Spectrum.vi"("Acquire"=w301, "Running"=w302, "ShutterOpen"=TRUE, "JYCCDLib.IJYCCDReqd"=w294) -> ("Raw Data"=w291:i32[][])  [unwired: 6 in, 1 out]
                                n147 = Index Array(array=w291, index (row)=0) -> (element=w290:i32[])  [unwired: 1 in]
                                n148 = local read "Wavelengths (nm)"() -> (w304:dbl[])
                                n149 = Increment(x=w309) -> (x+1=w295:i32)
                                n150 = Number To Decimal String(number=w295) -> (decimal integer string=w298:string)  [unwired: 1 in]
                                n151 = Concatenate Strings(w298, "/" ("string"), w299) -> (w297:string)
                                n152 = local write "CCD Current Rep."(w297) -> ()
                                n153 = Build Array (concatenate)(w290, w308) -> (w307:i32[][])
                                n154 = call "Symphony Average Spectra.vi"("Repetitions"=w295, "Raw Spectra"=w307) -> ("Raw Spectrum"=w306:dbl[])
                                n155 = local read "Start"() -> (w303:bool)
                                n156 = call "Spectrum Merge Wavelengths v10.5.0.vi"("Wavelengths (nm)"=w304, "Raw Spectrum"=w306) -> ("Spectrum-Cluster"=w305:T10)  [unwired: 1 out]
                                }
                                }
                                frame True {
                                # "simulate spectrum"
                                n157 = call "Mapping Simulated Spectrum v10.1.0.vi"() -> ("Simulated Spectrum"=w310:cluster{i32[], dbl[]}[])
                                }
                                }
                                n158 = local read "Target Position"() -> (w274:T7)
                                n159 = Index Array(array=w268, index=0 ("Index")) -> (element=w267:T11)
                                n160 = call "Mapping Merge Live Data v10.2.1.vi"("New Spectrum"=w267, "Target Position"=w274, "X in (1D)"=w282, "Y in (1D)"=w281, "L in (2D)"=w280, "I in (2D)"=w279, "Step Size"=w265) -> ("Live Data"=w273:dbl[][], "X out (1D)"=w276:dbl[], "Y out (1D)"=w275:dbl[], "L out (2D)"=w277:dbl[][], "I out (2D)"=w278:dbl[][])  [unwired: 4 in]
                                n161 = invoke class="VI Interface Type 0" method="Ctrl Val.Set"(reference=w284, "Control Name"="LiveData" ("Elementname"), "Value"=w273) -> ()  [unwired: 2 in, 5 out]
                                n162 = local write "Live Data"(w273) -> ()
                              }
                            }
                          }
                          frame #4 {
                            # "set new X"
                            n163 = Increment(x=w321) -> (x+1=w320:i32)
                            n164 = local read "Start"() -> (w314:bool)
                            n165 = Equal?(x=w319, y=w320) -> (x = y?=w311:bool)
                            n166 = Not(x=w314) -> (.not. x?=w313:bool)
                            n167 = Or(x=w311, y=w313) -> (x .or. y?=w312:bool)
                            n168 = case shown="True" w312 {
                              tunnel: w318 -> [w329 w337]
                              tunnel: [w328 w337] -> w315
                              tunnel: w317 -> [w327 _]
                              tunnel: w316 -> [w322 _]
                              frame False {
                                n169 = Unbundle By Name(w329) -> ("Drive X Position"=w330:dbl)
                                n170 = case shown="False" w327 {
                                tunnel: w330 -> [w333 w335]
                                tunnel: [w332 w336] -> w323
                                tunnel: w322 -> [w331 w334]
                                frame False {
                                n171 = Subtract(x=w333, y=w331) -> (x-y=w332:dbl)
                                }
                                frame True {
                                n172 = Add(x=w335, y=w334) -> (x+y=w336:dbl)
                                }
                                }
                                n173 = Divide(x=w323, y=w322) -> (x/y=w326:dbl)
                                n174 = Round To Nearest(number=w326) -> (nearest integer value=w325:dbl)
                                n175 = Multiply(x=w325, y=w322) -> (x*y=w324:dbl)
                                n176 = Bundle By Name(cluster=w329, "Drive X Position"=w324) -> (w328:T3)
                              }
                              frame True {
                              }
                            }
                            n177 = local write "Target Position"(w315) -> ()
                          }
                          frame #5 {
                            n178 = Tick Count (ms)() -> (millisecond timer value=w342:u32)
                            n179 = Subtract(x=w342, y=w341) -> (x-y=w344:u32)
                            n180 = Divide(x=w344, y=u32 1000) -> (x/y=w339:dbl)
                            n181 = Build Array (concatenate)(w340, w339) -> (w338:dbl[])
                          }
                        }
                        n182 = local read "Start"() -> (w199:bool)
                      }
                    }
                    frame #1 {
                      # "set new Y\nand move to new position"
                      n183 = Increment(x=w356) -> (x+1=w355:i32)
                      n184 = local read "Start"() -> (w346:bool)
                      n185 = Equal?(x=w354, y=w355) -> (x = y?=w348:bool)
                      n186 = local read "Simulate Drive"() -> (w349:bool)
                      n187 = Not(x=w346) -> (.not. x?=w347:bool)
                      n188 = Or(x=w348, y=w347) -> (x .or. y?=w345:bool)
                      n189 = case shown="False" w345 {
                        tunnel: w352 -> [w375 w376]
                        tunnel: [w374 w376] -> w350
                        tunnel: w353 -> [w369 _]
                        frame False {
                          n190 = Unbundle By Name(w375) -> ("Drive Y Position"=w373:dbl)
                          n191 = Add(x=w369, y=w373) -> (x+y=w370:dbl)
                          n192 = Divide(x=w370, y=w369) -> (x/y=w371:dbl)
                          n193 = Round To Nearest(number=w371) -> (nearest integer value=w372:dbl)
                          n194 = Multiply(x=w372, y=w369) -> (x*y=w368:dbl)
                          n195 = Bundle By Name(cluster=w375, "Drive Y Position"=w368) -> (w374:T3)
                        }
                        frame True {
                        }
                      }
                      n196 = case shown="False" w349 {
                        tunnel: w351 -> [w359 _]
                        tunnel: w350 -> [w358 _]
                        frame False {
                          n197 = flat-sequence {
                            tunnel: w359 -> [w364]
                            tunnel: w358 -> [w363]
                            tunnel: [w364] -> w360
                            tunnel: [w367] -> w357
                            tunnel: w360 -> [w366]
                            frame #0 {
                              n198 = Unbundle By Name(w363) -> ("Drive Y Position"=w362:dbl)
                              n199 = control-ref of="Objective Running"() -> (w365:refnum<vi>)
                              n200 = call "NPC3SG Move Axis To v10.6.1.vi"("Drive Visa Name"=w364, "Running"=w365, "Axis"=1, "Drive Set"=w362) -> ()  [unwired: 3 in, 1 out]
                            }
                            frame #1 {
                              n201 = call "NPC3SG Get Positions v10.6.1.vi"("Drive Visa Name"=w366) -> ("Drive Current Values"=w367:T3)  [unwired: 6 in]
                            }
                          }
                          n202 = global write "Global Variables.vi" "Global Piezo Position"(w357) -> ()
                          n203 = local write "Current Position"(w357) -> ()
                        }
                        frame True {
                        }
                      }
                      n204 = local write "Target Position"(w350) -> ()
                    }
                  }
                  n205 = local read "Start"() -> (w142:bool)
                }
              }
              frame #2 {
                # "conclude measurement"
                n206 = flat-sequence {
                  tunnel: w378 -> [w391]
                  tunnel: w377 -> [w390]
                  tunnel: w379 -> [w396]
                  frame #0 {
                    # "save data"
                    n207 = local read "Input Parameters"() -> (w384:T1)
                    n208 = global read "Global Variables.vi" "Global iHR Values"() -> (w387:T4)
                    n209 = global read "Global Variables.vi" "Global ITC Values"() -> (w388:T2)
                    n210 = local read "Spectra Params"() -> (w385:T5)
                    n211 = global read "Global Variables.vi" "Global CCD Temperature (C)"() -> (w386:dbl)
                    n212 = Unbundle By Name(w384) -> ("CCD Area"=w383:T6, "CCD Gain"=w381:u16, "CCD ADC"=w382:u16)
                    n213 = local read "Mapping Params"() -> (w380:T8)
                    n214 = call "Export_mappingFileName v10.5.1.vi"("ITC503 Current Values"=w388, "iHR Current Values"=w387, "Spectra Settings"=w385, "Mapping Parameters"=w380) -> ("Filename"=w394:string)  [unwired: 1 in]
                    "Filename" <- w394
                    n215 = local read "Live Data"() -> (w393:dbl[][])
                    n216 = Unbundle By Name(w380) -> ("Step Size"=w389:dbl)
                    n217 = call "Mapping Merge Real Positions v10.2.1.vi"("Live Data In"=w393, "X in (1D)"=w391, "Y in (1D)"=w390, "Step Size"=w389) -> ("Live Data Out"=w392:dbl[][])  [unwired: 11 in]
                    "Full Data" <- w392
                    n218 = call "Export_2DtoTxt v10.6.0.vi"("ITC503 Current Values"=w388, "iHR Current Values"=w387, "CCD Temperature"=w386, "CCD Area"=w383, "CCD ADC"=w382, "CCD Gain"=w381, "Export Type"="Mapping", "Spectra Settings"=w385, "Filename"=w394, "Data (2D)"=w392, "Mapping Parameters"=w380) -> ()  [unwired: 8 in, 1 out]
                  }
                  frame #1 {
                    # "reset indicators"
                    n219 = local write "Start"(FALSE ("Start")) -> ()
                    n220 = local write "CCD Current Rep."("0/0" ("CCD3000 Current Rep.")) -> ()
                    n221 = case shown="False" w396 {
                      frame False {
                        n222 = call "Video Toolset Stop.vi"() -> ()  [unwired: 3 in]
                      }
                      frame True {
                      }
                    }
                    n223 = property on="Measuring" class="Bool (strict)"("BoolText.Text"="" ("Boolescher Text.Text")) -> ()  [unwired: 2 in, 2 out]
                    n224 = property on="Measuring" class="Bool (strict)"("Blinking"=FALSE ("Measuring")) -> ()  [unwired: 2 in, 2 out]
                    n225 = global write "Global Variables.vi" "Mapping Running?"(FALSE ("Mapping Running?")) -> ()
                  }
                }
              }
            }
          }
        }
        n226 = local read "Exit"() -> (w40:bool)
      }
    }
    frame #2 {
      n227 = invoke class="VI Interface Type 0" method="Ctrl Val.Set"(reference=w403, "Control Name"="Exit" ("Elementname"), "Value"=TRUE) -> ()  [unwired: 2 in, 5 out]
      n228 = local read "AutoClose"() -> (w402:bool)
      n229 = flat-sequence {
        tunnel: w402 -> [w406]
        frame #0 {
          # "reset and close"
          n230 = control-ref of="Dieses VI"() -> (w409:refnum<vi>)
          n231 = global write "Global Variables.vi" "Mapping Open?"(FALSE ("Mapping Open?")) -> ()
          n232 = invoke class="VI" method="Default Vals.Reinit All"(reference=w409) -> (reference out=w407:refnum<vi>)  [unwired: 2 in, 2 out]
          n233 = property on="Measuring" class="Bool (strict)"("BoolText.Text"="" ("Boolescher Text.Text")) -> ()  [unwired: 2 in, 2 out]
          n234 = property class="App"() -> ("App.Kind"=w410:T12)  [unwired: 2 in, 2 out]
          n235 = case shown="\"invalid app kind\", Default" w410 {
            tunnel: w407 -> [w412 w414]
            tunnel: w406 -> [_ w413]
            frame "invalid app kind", Default {
              n236 = invoke on="Invoke Node" class="VI" method="FP.Close"(reference=w412) -> ()  [unwired: 2 in, 3 out]
            }
            frame "Development System" {
              n237 = case shown="True" w413 {
                tunnel: w414 -> [_ w415]
                frame False {
                }
                frame True {
                  n238 = invoke on="Invoke Node" class="VI" method="FP.Close"(reference=w415) -> ()  [unwired: 2 in, 3 out]
                }
              }
            }
          }
        }
      }
    }
  }
